vi "Init.vi"(8 "error in (no error)":errorcluster, 11 "VISA resource in":refnum<visa-resource-name>) -> (0 "error out":errorcluster, 3 "VISA resource out":refnum<visa-resource-name>)   [LabVIEW 2020, in "Omega Platinum Series Plugin.lvlib"]
uses:
  Omega Platinum Series Plugin.lvlib
  Typedefs/Init.vi States.ctl
  <instrlib>/RxnRover/OmegaPlatinumSeriesDriver/Omega Platinum Series.lvlib
panel:
  in  "Connect Btn":bool
  # "1. VISA Resource/Comm Port"
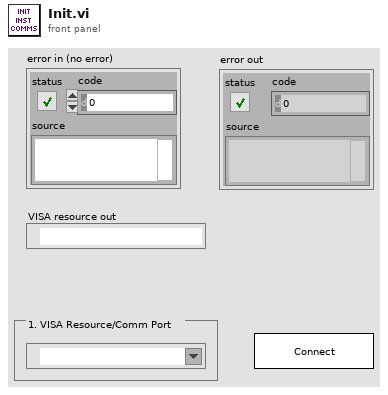
[diagram p1: front panel]
types:
  T1 = typedef "Omega Platinum Series Plugin.lvlib/Init.vi States.ctl" = enum16{"Waiting for connection", "Connecting", "Successful connection", "Failed to connect", "Closing"}
  T2 = enum32{"Invalid", "Standard", "Closed", "Hidden", "Minimized", "Maximized"}
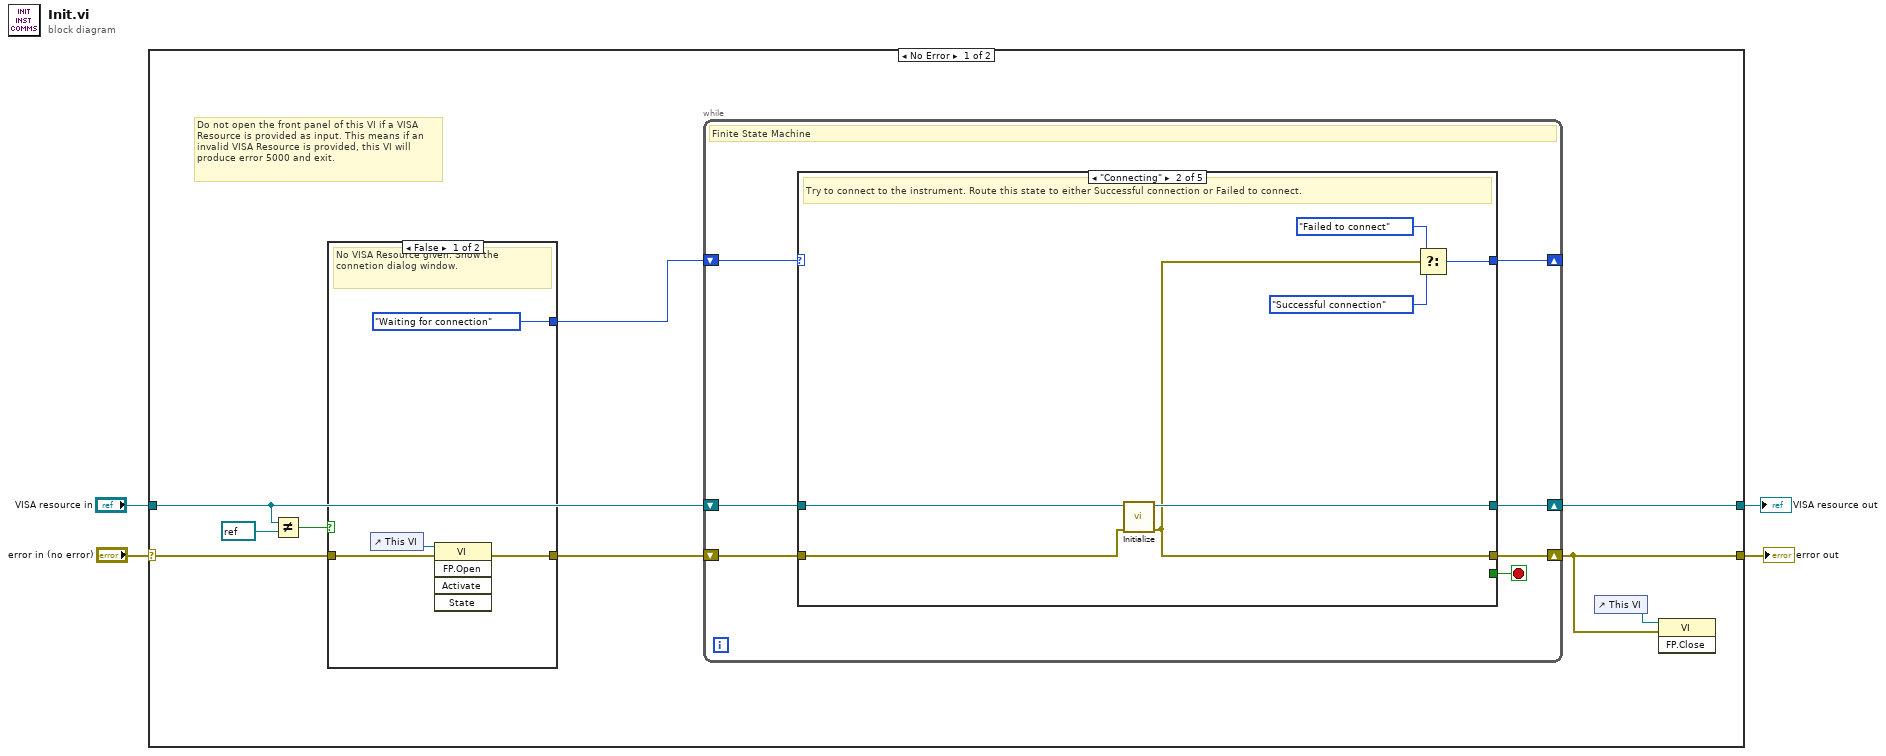
[diagram p0: block diagram]
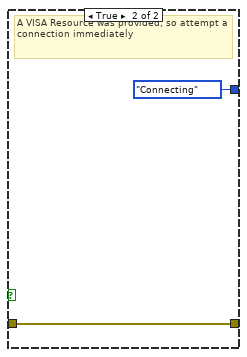
[diagram p2: hidden frame]
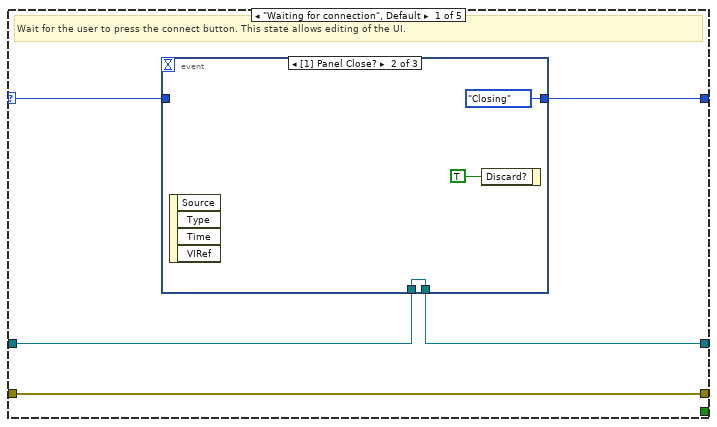
[diagram p3: hidden frame]
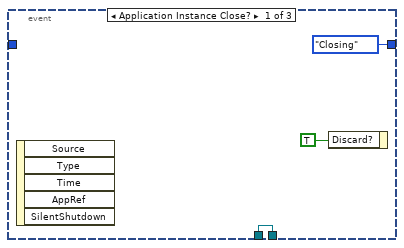
[diagram p4: hidden frame]
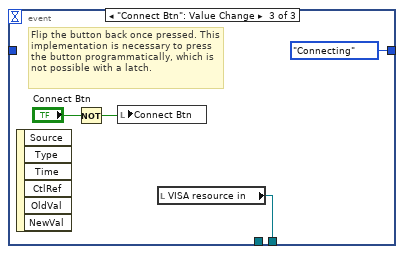
[diagram p5: hidden frame]
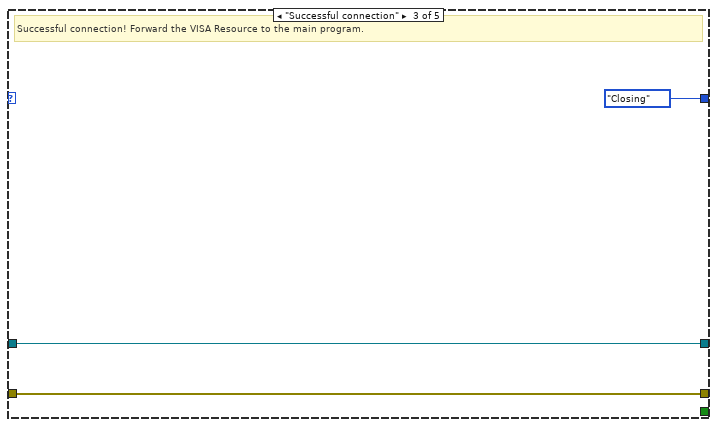
[diagram p6: hidden frame]
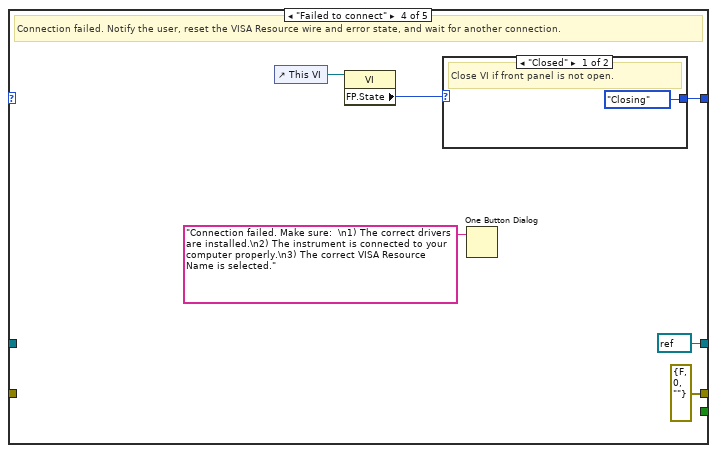
[diagram p7: hidden frame]
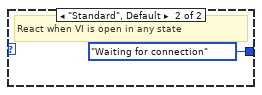
[diagram p8: hidden frame]
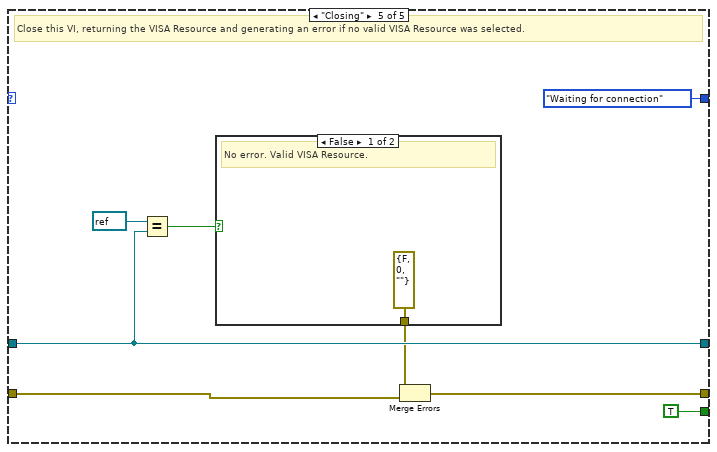
[diagram p9: hidden frame]
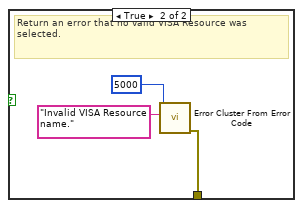
[diagram p10: hidden frame]
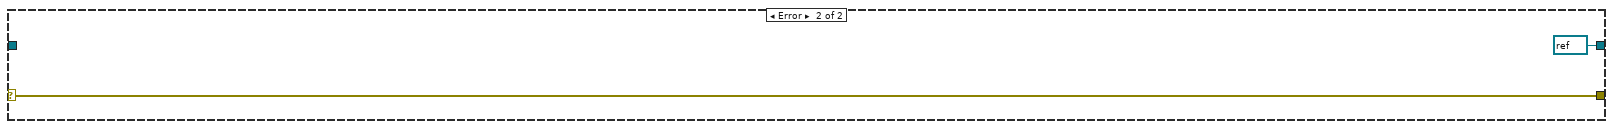
[diagram p11: hidden frame]
diagram:
  n1 = case shown="No Error" "error in (no error)" {
    selector: "error in (no error)" -> [w7 w73]
    tunnel: [w13 refnum<visa-resource-name> refnum ("VISA resource in")] -> w4
    tunnel: [w11 w73] -> w2
    tunnel: "VISA resource in" -> [w8 _]
    frame No Error {
      # "Do not open the front panel of this VI if a VISA Resource is provided as input. This means if an invalid VISA Resource is provided, this VI will produce error 5000 and exit."
      n2 = Not Equal?(x=w8, y=refnum<visa-resource-name> refnum ("x")) -> (x != y?=w10:bool)
      n3 = case shown="False" w10 {
        tunnel: w7 -> [w16 w19]
        tunnel: [w15 w19] -> w6
        tunnel: [Init.vi_States."Waiting for connection" Init.vi_States."Connecting"] -> w5
        frame False {
          # "No VISA Resource given. Show the connetion dialog window."
          n4 = control-ref of="This VI"() -> (w17:refnum<vi>)
          n5 = invoke class="VI" method="FP.Open"(reference=w17, error in=w16) -> (error out=w15:errorcluster)  [unwired: 3 in, 4 out]
        }
        frame True {
          # "A VISA Resource was provided, so attempt a connection immediately"
        }
      }
      n6 = while {
        shift-right: [w25] -> _
        shift-left: w5 -> [w26]
        shift-right: [w23] -> w13
        shift-left: w8 -> [w22]
        shift-right: [w20] -> w11
        shift-left: w6 -> [w21]
        stop <- w24 stop-if-true
        # "Finite State Machine"
        n7 = case shown="\"Connecting\"" w26 {
          selector: w26 -> [w31 _ _ _ _]
          tunnel: [w30 w48 Init.vi_States."Closing" w57 Init.vi_States."Waiting for connection"] -> w25
          tunnel: [_ _ _ _ TRUE] -> w24
          tunnel: [w27 w45 w50 refnum<visa-resource-name> refnum ("VISA resource in") w64] -> w23
          tunnel: w22 -> [w28 w42 w50 _ w64]
          tunnel: w21 -> [w29 w44 w49 _ w60]
          tunnel: [w29 w43 w49 errorcluster {"status"=FALSE, "code"=0, "source"=""} ("error IO") w61] -> w20
          frame "Waiting for connection", Default {
            # "Wait for the user to press the connect button. This state allows editing of the UI."
            n8 = event shown="[1] Panel Close?" {
              selector: _ -> [_ _ _]
              dyn-events: _ -> [_ _ _]
              timeout: _ -> [_ _ _]
              tunnel: [Init.vi_States."Closing" Init.vi_States."Closing" Init.vi_States."Connecting"] -> w30
              tunnel: w31 -> [_ _ _]
              tunnel: w28 -> [w32 w35 _]
              tunnel: [w32 w35 w38] -> w27
              event Application Instance Close? {
                n9 = event-data() -> ()  [unwired: 1 in, 5 out]
                n10 = event-data("Discard?"=TRUE) -> ()  [unwired: 1 in, 1 out]
              }
              event Panel Close? {
                n11 = event-data() -> ()  [unwired: 1 in, 4 out]
                n12 = event-data("Discard?"=TRUE) -> ()  [unwired: 1 in, 1 out]
              }
              event "Connect Btn": Value Change {
                # "Flip the button back once pressed. This implementation is necessary to press the button programmatically, which is not possible with a latch."
                n13 = event-data() -> ()  [unwired: 1 in, 6 out]
                n14 = Not(x="Connect Btn") -> (.not. x?=w39:bool)
                n15 = local write "Connect Btn"(w39) -> ()
                n16 = local read "VISA resource in"() -> (w38:refnum<visa-resource-name>)
              }
            }
          }
          frame "Connecting" {
            # "Try to connect to the instrument. Route this state to either Successful connection or Failed to connect."
            n17 = call <instrlib>:"Initialize.vi"("error in (no error)"=w44, "VISA resource name"=w42) -> ("error out"=w43:errorcluster, "VISA resource name out"=w45:refnum<visa-resource-name>)  [unwired: 7 in, 1 out]
            n18 = Select(t=Init.vi_States."Failed to connect", s=w43, f=Init.vi_States."Successful connection") -> (s? t:f=w48:T1)
          }
          frame "Successful connection" {
            # "Successful connection! Forward the VISA Resource to the main program."
          }
          frame "Failed to connect" {
            # "Connection failed. Notify the user, reset the VISA Resource wire and error state, and wait for another connection."
            n19 = control-ref of="This VI"() -> (w54:refnum<vi>)
            n20 = property class="VI"(reference=w54) -> ("FP.State"=w53:T2)  [unwired: 1 in, 2 out]
            n21 = case shown="\"Closed\"" w53 {
              tunnel: [Init.vi_States."Closing" Init.vi_States."Waiting for connection"] -> w57
              frame "Closed" {
                # "Close VI if front panel is not open."
              }
              frame "Standard", Default {
                # "React when VI is open in any state"
              }
            }
            n22 = One Button Dialog(message="Connection failed. Make sure:  \n1) The correct drivers are installed.\n2) The instrument is connected to your computer properly.\n3) The correct VISA Resource Name is selected.") -> ()  [unwired: 1 in, 1 out]
          }
          frame "Closing" {
            # "Close this VI, returning the VISA Resource and generating an error if no valid VISA Resource was selected."
            n23 = Equal?(x=refnum<visa-resource-name> refnum ("VISA resource in"), y=w64) -> (x = y?=w63:bool)
            n24 = case shown="False" w63 {
              tunnel: [errorcluster {"status"=FALSE, "code"=0, "source"=""} ("error out") w70] -> w62
              frame False {
                # "No error. Valid VISA Resource."
              }
              frame True {
                # "Return an error that no valid VISA Resource was selected."
                n25 = call <vilib>:"Error Cluster From Error Code.vi"("error message (\"\")"="Invalid VISA Resource name." ("error message (\"\")"), "error code (0)"=5000) -> ("error out"=w70:errorcluster)  [unwired: 7 in]
              }
            }
            n26 = Merge Errors(w62, w60) -> (w61:errorcluster)
          }
        }
      }
      n27 = control-ref of="This VI"() -> (w12:refnum<vi>)
      n28 = invoke class="VI" method="FP.Close"(reference=w12, error in=w11) -> ()  [unwired: 1 in, 3 out]
    }
    frame Error {
    }
  }
  "VISA resource out" <- w4
  "error out" <- w2
